vi "Draw Realtime if Ready.vi"(6 "3D":T2, 7 "Voltage Mapping":refnum<vi>, 8 "error in (no error)":errorcluster, 9 "Data Queue":refnum<queue>, 10 "3D Picture":refnum<vi>, 11 "Refnum in":T1) -> (0 "error out":errorcluster, 3 "Image out":T1)   [LabVIEW 2020]
doc: "This VI checks if the queue is not empty and sends the appropriate lithography points\nto be drawn."
uses:
  <vilib>/vision/Image Controls.llb/IMAQ Image.ctl
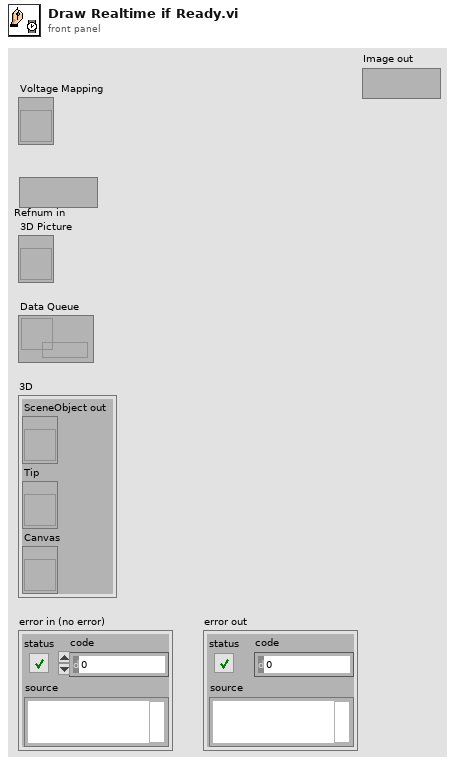
[diagram p1: front panel]
types:
  T1 = typedef "IMAQ Image.ctl" = refnum<image>
  T2 = cluster{"SceneObject out":refnum<vi>, "Tip":refnum<vi>, "Canvas":refnum<vi>}
  T3 = cluster{"X":dbl, "Y":dbl, "Speed":dbl, "Voltage":dbl}
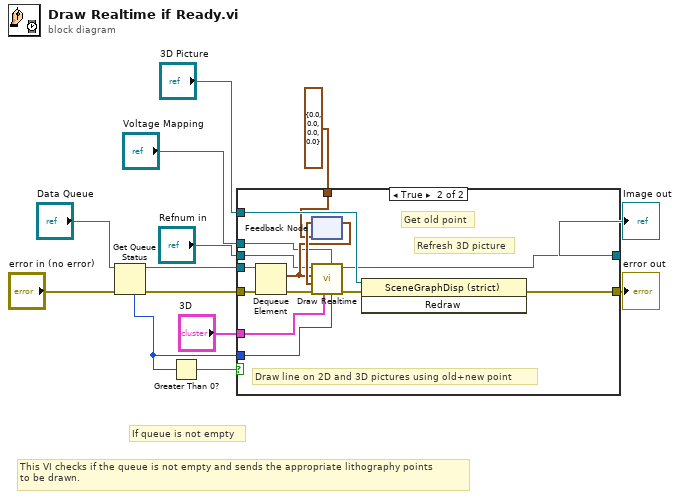
[diagram p0: block diagram]
diagram:
  # "This VI checks if the queue is not empty and sends the appropriate lithography points\nto be drawn."
  # "If queue is not empty"
  n1 = Get Queue Status(queue="Data Queue", error in (no error)="error in (no error)") -> (queue out=w6:refnum<queue>, error out=w5:errorcluster, # elements in queue=w10:i32)  [unwired: 1 in, 5 out]
  n2 = Greater Than 0?(x=w10) -> (x > 0?=w8:bool)
  n3 = case shown="True" w8 {
    tunnel: [w15 w27] -> w9
    tunnel: w6 -> [_ w26]
    tunnel: w5 -> [w15 w25]
    tunnel: "3D" -> [_ w23]
    tunnel: w10 -> [_ w22]
    tunnel: "Voltage Mapping" -> [_ w21]
    tunnel: "3D Picture" -> [_ w20]
    tunnel: "Refnum in" -> [w14 w19]
    tunnel: [w14 w17] -> w2
    tunnel: T3 {"X"=0.0, "Y"=0.0, "Speed"=0.0, "Voltage"=0.0} ("Litho Point") -> [_ w16]
    frame False {
    }
    frame True {
      # "Get old point"
      # "Draw line on 2D and 3D pictures using old+new point"
      # "Refresh 3D picture"
      n4 = Dequeue Element(queue=w26, error in (no error)=w25) -> (element=w24:T3, error out=w29:errorcluster)  [unwired: 1 in, 2 out]
      n5 = feedback #1(w16) -> (w28:T3)
      n6 = feedback-in #1(w24) -> ()
      n7 = call "Draw Realtime.vi"("Queue Items"=w22, "ColorRamp in"=w21, "3D"=w23, "error in (no error)"=w29, "Litho Point Old"=w28, "Litho Point"=w24, "Image in"=w19) -> ("error out"=w18:errorcluster, "Image out"=w17:T1)  [unwired: 3 in]
      n8 = invoke class="SceneGraphDisp (strict)" method="Redraw"(reference=w20, error in=w18) -> (error out=w27:errorcluster)  [unwired: 1 in, 2 out]
    }
  }
  "error out" <- w9
  "Image out" <- w2
